vi "Utility Create Public Directory.vi"(8 "error in (no error)":errorcluster, 11 "reference":refnum<vi>) -> (0 "error out":errorcluster, 3 "PATH":path)   [LabVIEW 2015]
uses:
  <vilib>/Utility/sysdir.llb/System Directory Type.ctl
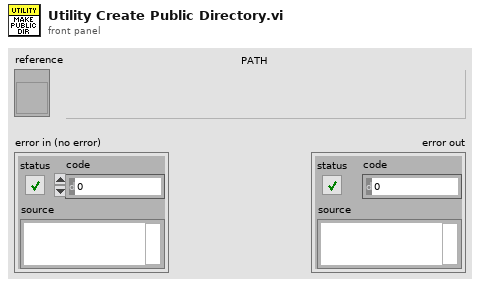
[diagram p1: front panel]
types:
  T1 = typedef "System Directory Type.ctl" = i32
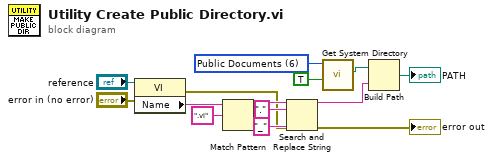
[diagram p0: block diagram]
diagram:
  w14 = T1 6 items=["User Home"=0, "User Desktop"=1, "User Documents"=2, "User Application Data"=3, "User Preferences"=4, "User Temporary"=5, "Public Documents"=6, "Public Application Data"=7, "Public Preferences"=8, "Public Cache"=13, "System Core Libraries"=9, "System Installed Libraries"=10, "Application Files"=11, "Boot Volume Root"=12] ("system directory type")
  n1 = property class="VI"(reference="reference", error in="error in (no error)") -> (error out=w2:errorcluster, "Name"=w6:string)  [unwired: 1 out]
  n2 = Match Pattern(string=w6, regular expression=".vi") -> (before substring=w8:string)  [unwired: 1 in, 3 out]
  n3 = Search and Replace String(input string=w8, search string=".", replace string="_" ("replace string (\"\")"), error in=w2) -> (result string=w7:string, error out=→"error out":errorcluster)  [unwired: 4 in, 2 out]
  n4 = call <vilib>:"Get System Directory.vi"("create directory if not found? (F)"=TRUE, "system directory type"=w14) -> ("system directory"=w12:path)  [unwired: 9 in]
  n5 = Build Path(base path=w12, name or relative path=w7) -> (appended path=→"PATH":path)
